vi "Draw overlay lines.vi"(8 "error in (no error)":errorcluster, 10 "IMAQ reference":T1, 11 "DAQOrcaFlash in":refnum<class "DAQOrcaFlash.lvclass">) -> (0 "error out":errorcluster, 2 "IMAQ reference out":T1, 3 "DAQOrcaFlash out":refnum<class "DAQOrcaFlash.lvclass">)   [LabVIEW 2012, in "DAQOrcaFlash.lvclass"]
uses:
  DAQOrcaFlash.lvclass
  <vilib>/vision/Image Controls.llb/IMAQ Image.ctl
  DAQOrcaFlash.lvclass/DAQOrcaFlash.ctl
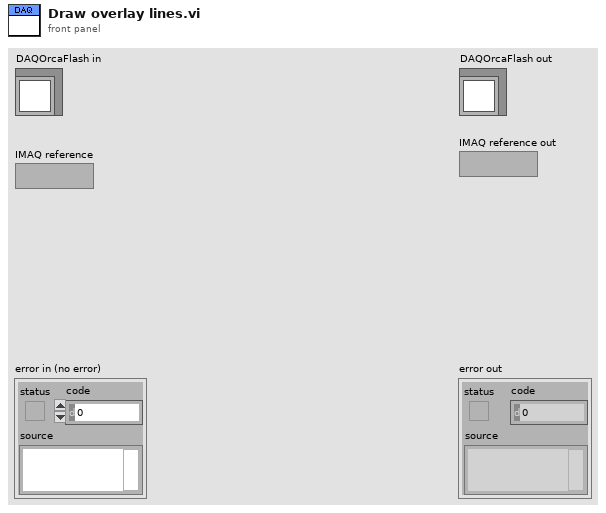
[diagram p1: front panel]
types:
  T1 = typedef "IMAQ Image.ctl" = refnum<image>
  T2 = typedef "DAQOrcaFlash.lvclass/visualisation_line_cluster.ctl" = cluster{"direction":enum16{"horizontal", "vertical"}, "position":i32}
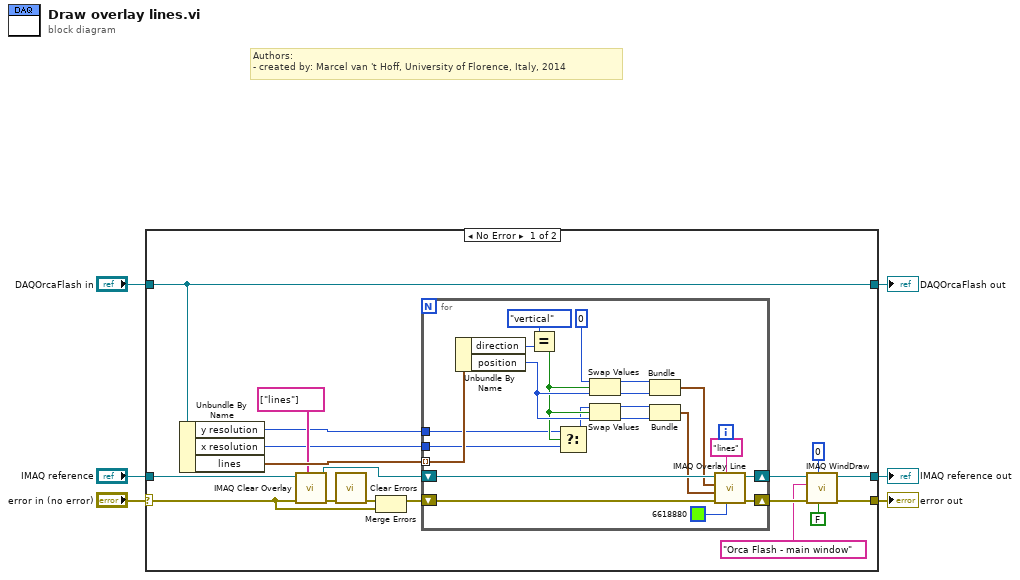
[diagram p0: block diagram]
diagram:
  # "Authors: \n- created by: Marcel van 't Hoff, University of Florence, Italy, 2014"
  n1 = case shown="No Error" "error in (no error)" {
    selector: "error in (no error)" -> [w20 w48]
    tunnel: [w13 w48] -> w5
    tunnel: [w8 w47] -> w3
    tunnel: "DAQOrcaFlash in" -> [w8 w47]
    tunnel: "IMAQ reference" -> [w9 w46]
    tunnel: [w7 w46] -> w1
    frame No Error {
      n2 = Unbundle By Name(w8) -> ("y resolution"=w17:i32, "x resolution"=w16:i32, "lines"=w24:T2[])
      n3 = call "IMAQ Clear Overlay"("Groups"=string[] ["lines"], "error in (no error)"=w20, "Image"=w9) -> ("error out"=w22:errorcluster, "Image Out"=w21:T1)  [unwired: 7 in]
      n4 = call <vilib>:"Clear Errors.vi"("error in (no error)"=w22) -> ("error out"=w19:errorcluster)  [unwired: 6 in]
      n5 = Merge Errors(w19, w20) -> (w18:errorcluster)
      n6 = for {
        shift-right: [w43] -> w14
        shift-left: w18 -> [w44]
        tunnel: w24 -> [w41] mode=indexing
        tunnel: w17 -> [w26]
        shift-right: [w29] -> w15
        shift-left: w21 -> [w45]
        tunnel: w16 -> [w27]
        n7 = Unbundle By Name(w41) -> ("direction"=w40:enum16{"horizontal", "vertical"}, "position"=w33:i32)
        n8 = Equal?(x=enum16{"horizontal", "vertical"}."vertical" ("direction"), y=w40) -> (x = y?=w28:bool)
        n9 = Select(t=w26, s=w28, f=w27) -> (s? t:f=w25:i32)
        n10 = Swap Values(12:0 ("y"), 13:w28, 14:w33) -> (1:w37:i32, 3:w32:i32)
        n11 = Swap Values(12:w25, 13:w28, 14:w33) -> (1:w31:i32, 3:w34:i32)
        n12 = Bundle(w37, w32) -> (w36:cluster{i32, i32})  [unwired: 1 in]
        n13 = Bundle(w31, w34) -> (w35:cluster{i32, i32})  [unwired: 1 in]
        n14 = call "IMAQ Overlay Line"("Color"=u32 6618880, "Group"="lines", "error in (no error)"=w44, "End Point"=w35, "Start Point"=w36, "Image"=w45) -> ("error out"=w43:errorcluster, "Image Out"=w29:T1)  [unwired: 4 in]
      }
      n15 = call "IMAQ WindDraw"("Resize to Image Size? (Y)"=FALSE, "Window Number (0...15)"=0, "error in (no error)"=w14, "Title"="Orca Flash - main window", "Image"=w15) -> ("error out"=w13:errorcluster, "Image Out (duplicate)"=w7:T1)  [unwired: 5 in]
    }
    frame Error {
    }
  }
  "error out" <- w5
  "DAQOrcaFlash out" <- w3
  "IMAQ reference out" <- w1
